vi "Miscellaneous_Test.vi"(1 "Joystick_Out":T1) -> ()   [LabVIEW 2020]
uses:
  Utility VIs/Joystick_Controls.ctl
  Globals/Calibration_And_Constant_Globals.vi
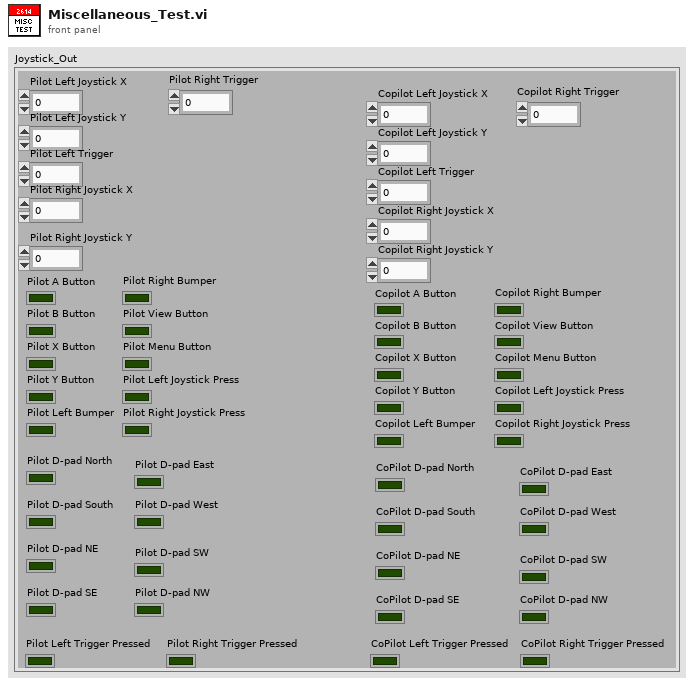
[diagram p1: front panel]
types:
  T1 = typedef "Joystick_Controls.ctl" = cluster{"Pilot Left Joystick X":dbl, "Pilot Left Joystick Y":dbl, "Pilot A Button":bool, "Pilot B Button":bool, "Pilot X Button":bool, "Pilot Y Button":bool, "Pilot Left Bumper":bool, "Pilot Right Bumper":bool, "Pilot View Button":bool, "Pilot Menu Button":bool, "Pilot Left Joystick Press":bool, "Pilot Right Joystick Press":bool, "Pilot Left Trigger":dbl, "Pilot Right Joystick X":dbl, "Pilot Right Joystick Y":dbl, "Pilot Right Trigger":dbl, "Copilot Left Joystick X":dbl, "Copilot Left Joystick Y":dbl, "Copilot A Button":bool, "Copilot B Button":bool, "Copilot X Button":bool, "Copilot Y Button":bool, "Copilot Left Bumper":bool, "Copilot Right Bumper":bool, "Copilot View Button":bool, "Copilot Menu Button":bool, "Copilot Left Joystick Press":bool, "Copilot Right Joystick Press":bool, "Copilot Left Trigger":dbl, "Copilot Right Joystick X":dbl, "Copilot Right Joystick Y":dbl, "Copilot Right Trigger":dbl, "Pilot D-pad North":bool, "Pilot D-pad South":bool, "Pilot D-pad East":bool, "Pilot D-pad West":bool, "Pilot D-pad NE ":bool, "Pilot D-pad SE":bool, "Pilot D-pad SW":bool, "Pilot D-pad NW":bool, "CoPilot D-pad North":bool, "CoPilot D-pad South":bool, "CoPilot D-pad East":bool, "CoPilot D-pad West":bool, "CoPilot D-pad NE":bool, "CoPilot D-pad SE":bool, "CoPilot D-pad SW":bool, "CoPilot D-pad NW":bool, "Pilot Left Trigger Pressed":bool, "Pilot Right Trigger Pressed":bool, "CoPilot Left Trigger Pressed":bool, "CoPilot Right Trigger Pressed":bool}
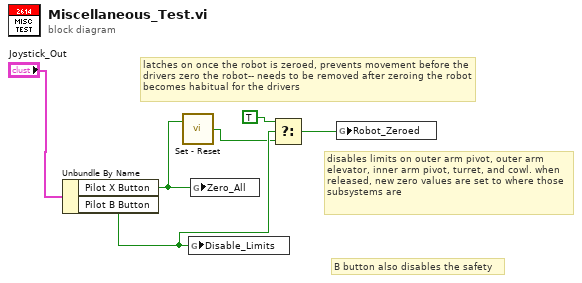
[diagram p0: block diagram]
diagram:
  # "B button also disables the safety"
  # "latches on once the robot is zeroed, prevents movement before the drivers zero the robot-- needs to be removed after zeroing the robot becomes habitual for the drivers"
  # "disables limits on outer arm pivot, outer arm elevator, inner arm pivot, turret, and cowl. when released, new zero values are set to where those subsystems are"
  n1 = Unbundle By Name("Joystick_Out") -> ("Pilot X Button"=w6:bool, "Pilot B Button"=w4:bool)
  n2 = call "Set - Reset.vi"("Set"=w6) -> ("Output"=w2:bool)  [unwired: 1 in]
  n3 = global write "Calibration_And_Constant_Globals.vi" "Disable_Limits"(w4) -> ()
  n4 = global write "Calibration_And_Constant_Globals.vi" "Zero_All"(w6) -> ()
  n5 = Select(t=TRUE ("Pilot B Button"), s=w4, f=w2) -> (s? t:f=w1:bool)
  n6 = global write "Calibration_And_Constant_Globals.vi" "Robot_Zeroed"(w1) -> ()
